vi "NS Writer.vi"() -> ()   [LabVIEW 2014]
uses:
  <resource>/objmgr/ni.dex.rc
panel:
  in  "Frequency":bool
  in  "Stop":bool
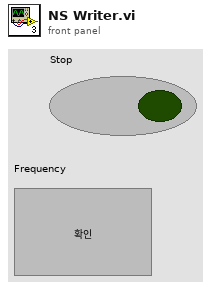
[diagram p1: front panel]
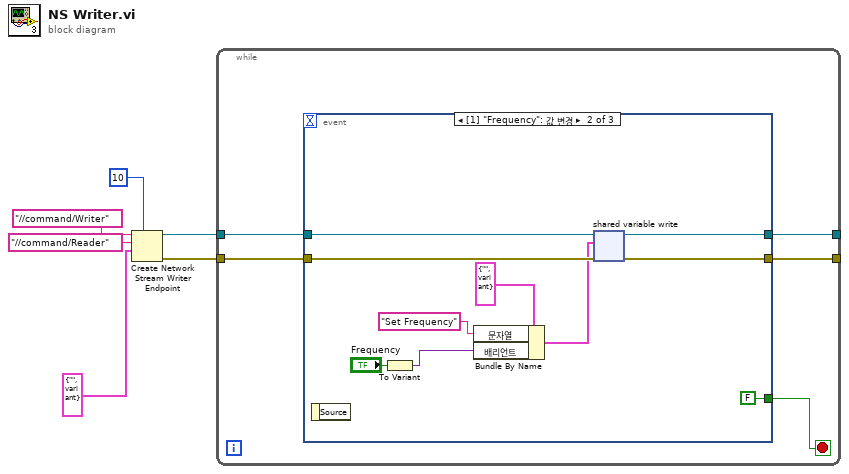
[diagram p0: block diagram]
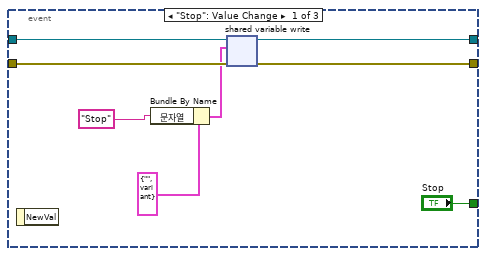
[diagram p2: hidden frame]
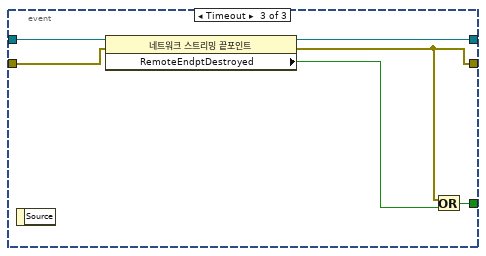
[diagram p3: hidden frame]
diagram:
  n1 = Create Network Stream Writer Endpoint(7:10 ("발신자 버퍼 크기"), 9:cluster{"문자열":string, "배리언트":variant} {"문자열"="", "배리언트"=variant} ("클러스터"), 10:"//command/Reader" ("수신자 URL"), 11:"//command/Writer" ("발신자 이름")) -> (0:w5:errorcluster, 3:w6:refnum<k21>)  [unwired: 3 in]
  n2 = while {
    tunnel: w6 -> [w10]
    tunnel: w5 -> [w9]
    tunnel: [w8] -> _
    tunnel: [w7] -> _
    stop <- w11 stop-if-true
    n3 = event shown="[1] \"Frequency\": 값 변경" {
      selector: _ -> [_ _ _]
      dyn-events: _ -> [_ _ _]
      timeout: _ -> [_ _ _]
      tunnel: ["Stop" FALSE ("Stop") w32] -> w11
      tunnel: w10 -> [w18 w23 w35]
      tunnel: w9 -> [w17 w22 w33]
      tunnel: [w13 w25 w34] -> w8
      tunnel: [w12 w24 w31] -> w7
      event "Stop": Value Change {
        n4 = event-data() -> ()  [unwired: 1 in, 1 out]
        n5 = Bundle By Name(cluster=cluster{"문자열":string, "배리언트":variant} {"문자열"="", "배리언트"=variant} ("클러스터"), "문자열"="Stop") -> (w14:cluster{"문자열":string, "배리언트":variant})
        n6 = shared-variable-write(w18, w17, w14) -> (w13:refnum<k21>, w12:errorcluster)  [unwired: 1 in, 1 out]
      }
      event "Frequency": Value Change {
        n7 = event-data() -> ()  [unwired: 1 in, 1 out]
        n8 = To Variant(anything="Frequency") -> (Variant=w26:variant)
        n9 = Bundle By Name(cluster=cluster{"문자열":string, "배리언트":variant} {"문자열"="", "배리언트"=variant} ("클러스터"), "문자열"="Set Frequency", "배리언트"=w26) -> (w21:cluster{"문자열":string, "배리언트":variant})
        n10 = shared-variable-write(w23, w22, w21) -> (w25:refnum<k21>, w24:errorcluster)  [unwired: 1 in, 1 out]
      }
      event Timeout {
        n11 = event-data() -> ()  [unwired: 1 in, 1 out]
        n12 = property on="프로퍼티 노드" class="네트워크 스트리밍 끝포인트"(reference=w35, error in=w33) -> (reference out=w34:refnum<k21>, error out=w31:errorcluster, "RemoteEndptDestroyed"=w30:bool)
        n13 = Or(x=w31, y=w30) -> (x .or. y?=w32:bool)
      }
    }
  }
